vi "Settings.vi"(8 "error in (no error)":errorcluster, 10 "variant":variant, 11 "Module":refnum<class "ModuleAdmin.lvclass">) -> (0 "error out":errorcluster)   [LabVIEW 2018, in "AcPwrPlugins.lvlib"]
uses:
  AcPwrPlugins.lvlib
  <userlib>/NIST/ModuleAdminLib/ModuleAdmin/ModuleAdmin.lvclass
  clEventType.ctl
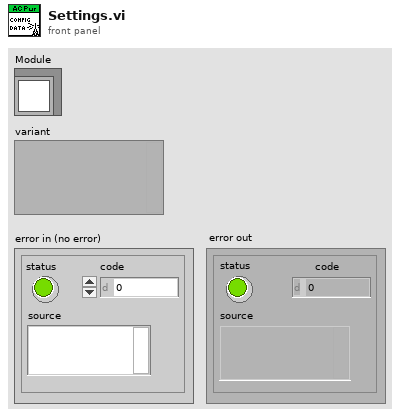
[diagram p1: front panel]
types:
  T1 = typedef "clBroadcastEvents.ctl" = cluster{"DidInit":refnum<user-event>, "StatusUpdate":refnum<user-event>, "ErrorReport":refnum<user-event>, "DidStop":refnum<user-event>, "PathToINI":refnum<user-event>, "Measurements":refnum<user-event>, "LoadConfigFile":refnum<user-event>, "GetSettings":refnum<user-event>, "SetSettings":refnum<user-event>, "GetType&ID":refnum<user-event>, "GotSettings":refnum<user-event>}
  T2 = typedef "clEventType.ctl" = cluster{"ModuleID":i32, "Data":variant}
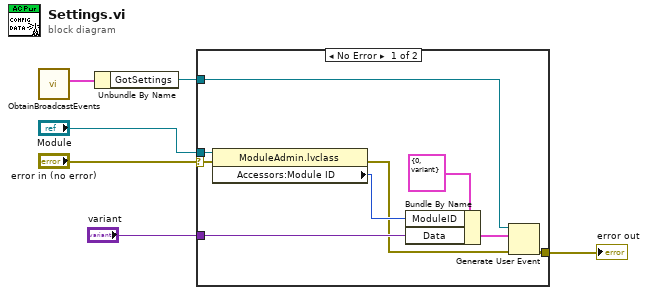
[diagram p0: block diagram]
diagram:
  n1 = call "ObtainBroadcastEvents.vi"() -> ("clAcPwrEvents"=w3:T1)  [unwired: 10 in, 1 out]
  n2 = Unbundle By Name(w3) -> ("GotSettings"=w2:refnum<user-event>)
  n3 = case shown="No Error" "error in (no error)" {
    selector: "error in (no error)" -> [w15 w16]
    tunnel: "Module" -> [w14 _]
    tunnel: [w13 w16] -> w4
    tunnel: w2 -> [w12 _]
    tunnel: "variant" -> [w11 _]
    frame No Error {
      n4 = property class="ModuleAdmin.lvclass"(reference=w14, error in=w15) -> (error out=w9:errorcluster, "Accessors:Module ID"=w10:i32)  [unwired: 1 out]
      n5 = Bundle By Name(cluster=T2 {"ModuleID"=0, "Data"=variant} ("clEventType"), "ModuleID"=w10, "Data"=w11) -> (w7:T2)
      n6 = Generate User Event(user event=w12, event data cluster=w7, error in=w9) -> (error out=w13:errorcluster)  [unwired: 1 in, 1 out]
    }
    frame Error {
    }
  }
  "error out" <- w4
